vi "Log Messages.vi"(8 "error in (no error)":errorcluster, 10 "Actor to Log":refnum<class "Message Enqueuer.lvclass">, 11 "Monitor in":refnum<class "Classic Monitor.lvclass">) -> (0 "error out":errorcluster, 3 "Monitor out":refnum<class "Classic Monitor.lvclass">)   [LabVIEW 2020, in "Monitored Actor.lvlib" / "Classic Monitor.lvclass"]
doc: "Starts message logging on the specified actor\n\nCopyright: MGI 2016\nAuthor: Derek Trepanier"
uses:
  <vilib>/MGI/Monitored Actor/Classic Monitor/Monitor/Monitor Actor/Classic Monitor.lvclass
  C:/Program Files/National Instruments/LabVIEW 2020/vi.lib/MGI/Monitored Actor/Actor Monitor/Actor Monitor/Actor Monitor.lvclass
  C:/Program Files/National Instruments/LabVIEW 2020/vi.lib/ActorFramework/Actor/Actor.lvclass
  <vilib>/ActorFramework/Message Enqueuer/Message Enqueuer.lvclass
  <vilib>/MGI/Monitored Actor/Actor Monitor/Actor Monitor/Actor Monitor.lvclass/Actor Monitor.ctl
  <vilib>/MGI/Monitored Actor/Classic Monitor/Monitor/Monitor Actor/Classic Monitor.lvclass/Classic Monitor.ctl
  <vilib>/MGI/Monitored Actor/Classic Monitor/Logger/Classic Logger Actor/Classic Logger.lvclass
  <vilib>/ActorFramework/Actor/Actor.lvclass/Actor.ctl
  <vilib>/ActorFramework/Message Enqueuer/Message Enqueuer.lvclass/Message Enqueuer.ctl
  <vilib>/ActorFramework/Message Enqueuer/Init from Existing Queue.vi
  <vilib>/MGI/Monitored Actor/Monitor Data/Monitor Data.lvclass
  <vilib>/MGI/Monitored Actor/Actor Monitor/Actor Monitor/Actor Monitor.lvclass
  <vilib>/ActorFramework/Actor/Actor.lvclass
  <vilib>/MGI/Monitored Actor/Classic Monitor/Logger/Classic Logger Messages/Start Logging Msg/Start Logging Msg.lvclass
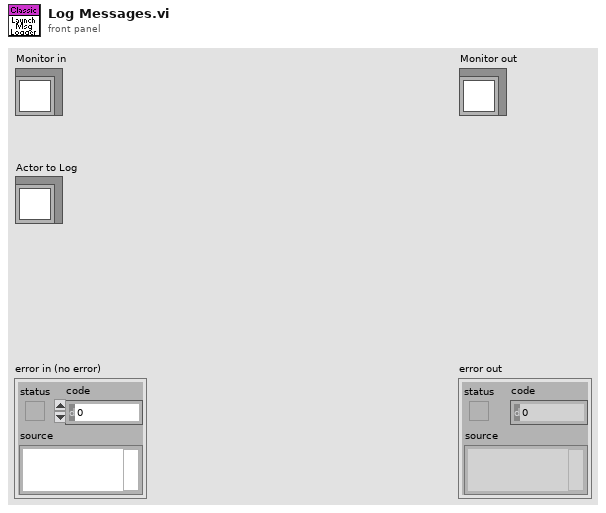
[diagram p1: front panel]
types:
  T1 = typedef "Monitor Data.lvclass/Actor Data.ctl" = cluster{"Actor Type":string, "Actor Core VI":string, "Self":refnum<class "Message Enqueuer.lvclass">, "Caller":refnum<class "Message Enqueuer.lvclass">, "Actor Label":string, "Last Ping":dbl}
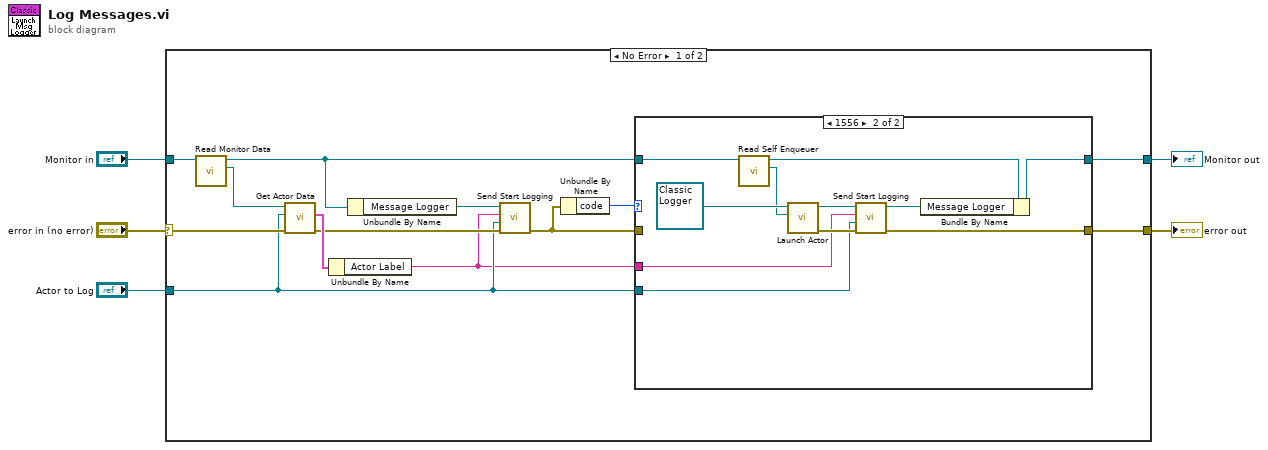
[diagram p0: block diagram]
diagram:
  n1 = case shown="No Error" "error in (no error)" {
    selector: "error in (no error)" -> [w15 w32]
    tunnel: [w16 w32] -> w4
    tunnel: [w18 w31] -> w2
    tunnel: "Monitor in" -> [w17 w31]
    tunnel: "Actor to Log" -> [w7 _]
    frame No Error {
      n2 = call <vilib>:"Read Monitor Data.vi"("Actor Monitor New in"=w17) -> ("Monitored Actor.lvlib:Monitor Data.lvclass"=w13:refnum<class "Monitor Data.lvclass">, "Actor Monitor New out"=w14:refnum<class "Classic Monitor.lvclass">)  [unwired: 8 in, 1 out]
      n3 = call <vilib>:"Get Actor Data.vi"("error in (no error)"=w15, "Actor's Self Q"=w7, "Monitor Data in"=w13) -> ("error out"=w9:errorcluster, "Actor Data"=w12:T1)  [unwired: 4 in, 3 out]
      n4 = Unbundle By Name(w12) -> ("Actor Label"=w6:string)
      n5 = Unbundle By Name(w14) -> ("Message Logger"=w10:refnum<class "Message Enqueuer.lvclass">)
      n6 = call <vilib>:"Send Start Logging.vi"("error in (no error)"=w9, "Actor to Log"=w7, "Label"=w6, "Message Enqueuer in"=w10) -> ("error out"=w8:errorcluster)  [unwired: 6 in, 1 out]
      n7 = Unbundle By Name(w8) -> ("code"=w11:i32)
      n8 = case shown="1556" w11 {
        tunnel: [w20 w30] -> w18
        tunnel: w14 -> [w20 w28]
        tunnel: w7 -> [_ w22]
        tunnel: w6 -> [_ w21]
        tunnel: [w19 w23] -> w16
        tunnel: w8 -> [w19 _]
        frame Default {
        }
        frame 1556 {
          n9 = call <vilib>:"Read Self Enqueuer.vi"("Actor"=w28) -> ("Self Enqueuer"=w27:refnum<class "Message Enqueuer.lvclass">)  [unwired: 10 in]
          n10 = call <vilib>:"Launch Actor.vi"("Actor-to-Caller Enqueuer"=w27, "Actor"=refnum<class "Classic Logger.lvclass"> refnum ("Classic Monitor.lvlib:Message Logger.lvclass")) -> ("error out"=w26:errorcluster, "Caller-To-Actor Enqueuer"=w25:refnum<class "Message Enqueuer.lvclass">)  [unwired: 8 in]
          n11 = call <vilib>:"Send Start Logging.vi"("error in (no error)"=w26, "Actor to Log"=w22, "Label"=w21, "Message Enqueuer in"=w25) -> ("error out"=w23:errorcluster, "Message Enqueuer out"=w24:refnum<class "Message Enqueuer.lvclass">)  [unwired: 6 in]
          n12 = Bundle By Name(cluster=w28, "Message Logger"=w24) -> (w30:refnum<class "Classic Monitor.lvclass">)
        }
      }
    }
    frame Error {
    }
  }
  "error out" <- w4
  "Monitor out" <- w2
